vi "BasicExampleWithIFw.vi"() -> ()   [LabVIEW 2015]
uses:
  QuadEnc/Output.ctl
  <vilib>/Platform/TimedLoop/XDataNode/timing_clust.ctl
  <vilib>/Platform/TimedLoop/XDataNode/nitl_modes.ctl
  <vilib>/Platform/TimedLoop/XDataNode/wakeup.ctl
  <vilib>/rvi/Emulation/niFpgaSctlEmulationGetInTimedLoop.vi
  <vilib>/rvi/Emulation/niFpgaEmulationReportErrorSimple.vi
  <vilib>/rvi/Emulation/niFpgaGetClockAttributes.vi
  <vilib>/rvi/Emulation/niFpgaCriticalErrorInLSC.vi
  <vilib>/rvi/eio/common/nirviEmuTemplateMethod_errors.vi
  <vilib>/Platform/TimedLoop/XDataNode/XDataNode.xnode
  <vilib>/eio/EIONode/EIONode.xnode
  <instrlib>/_niInstr/Instruction Framework/v1/FPGA/Top Level Bus/Register Configuration/Register Configuration.lvclass
  <vilib>/Platform/TimedLoop/XDataNode/XDNodeRunTimeDep.lvlib
  QuadEnc/AddressSpace.lvclass
  QuadEnc/QuadEnc.lvlib
  <instrlib>/_niInstr/FIFO Register Bus/v1/FPGA/niInstr FIFO Register Bus v1 FPGA.lvclass
panel:
  in  "fifo reg bus ctrl 0":u32
  out "fifo reg bus status 0":u32
  out "fifo reg bus data 0":u64
  in  "reset":bool
  out "AbsPosition":i32
  out "RevPosition":i32
  out "CW_direction":bool
  out "Output":T1
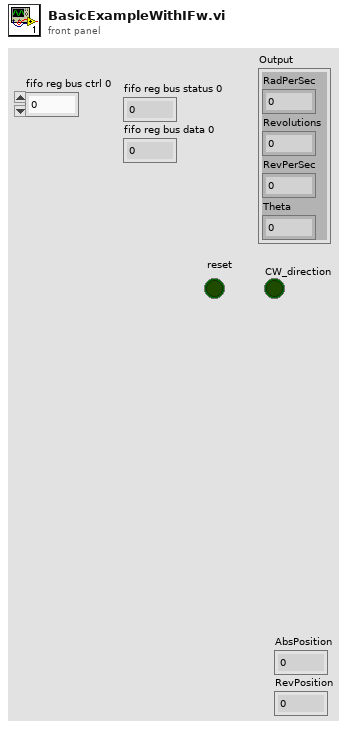
[diagram p1: front panel]
types:
  T1 = typedef "QuadEnc.lvlib/Output.ctl" = cluster{"RadPerSec":sgl, "Revolutions":sgl, "RevPerSec":sgl, "Theta":sgl}
  T2 = typedef "XDNodeRunTimeDep.lvlib/timing_clust.ctl" = cluster{"Expected End [f-1]":u64, "Actual End [f-1]":u64, "Finished Late? [f-1]":bool, "Expected End [i-1]":u64, "Actual End [i-1]":u64, "Finished Late? [i-1]":bool, "Expected Start [i]":u64, "Actual Start [i]":u64, "Expected Start [f]":u64, "Actual Start [f]":u64, "Source Name":string, "Structure Name":string, "Period":i64, "Deadline":i64, "Offset":i64, "Start":i64, "Priority":i32, "Timeout":i32, "Mode":T3, "Wakeup Reason":T4, "Error":errorcluster, "Source Type":string, "Secondary Source Type":string, "Global End Time":u64, "Global Start Time":u64, "Frame Duration":u64, "Iteration Duration":u64, "Assigned CPU":i32, "I/O Scan Engine Mode":u32}
  T3 = typedef "XDNodeRunTimeDep.lvlib/nitl_modes.ctl" = enum32{"No Change", "Process missed periods, maintain original phase", "Discard missed periods, maintain original phase", "Process missed periods, ignore original phase", "Discard missed periods, ignore original phase"}
  T4 = typedef "XDNodeRunTimeDep.lvlib/wakeup.ctl" = enum32{"Normal", "Aborted", "Asynchronous wakeup", "Timing source error", "Timed loop error", "Timeout"}
  T5 = typedef "QuadEnc.lvlib/Parameters.ctl" = cluster{"ReversePolarity":refnum<k21>, "dTPerSec":refnum<k21>, "RevPerPulse":refnum<k21>, "dT":refnum<k21>}
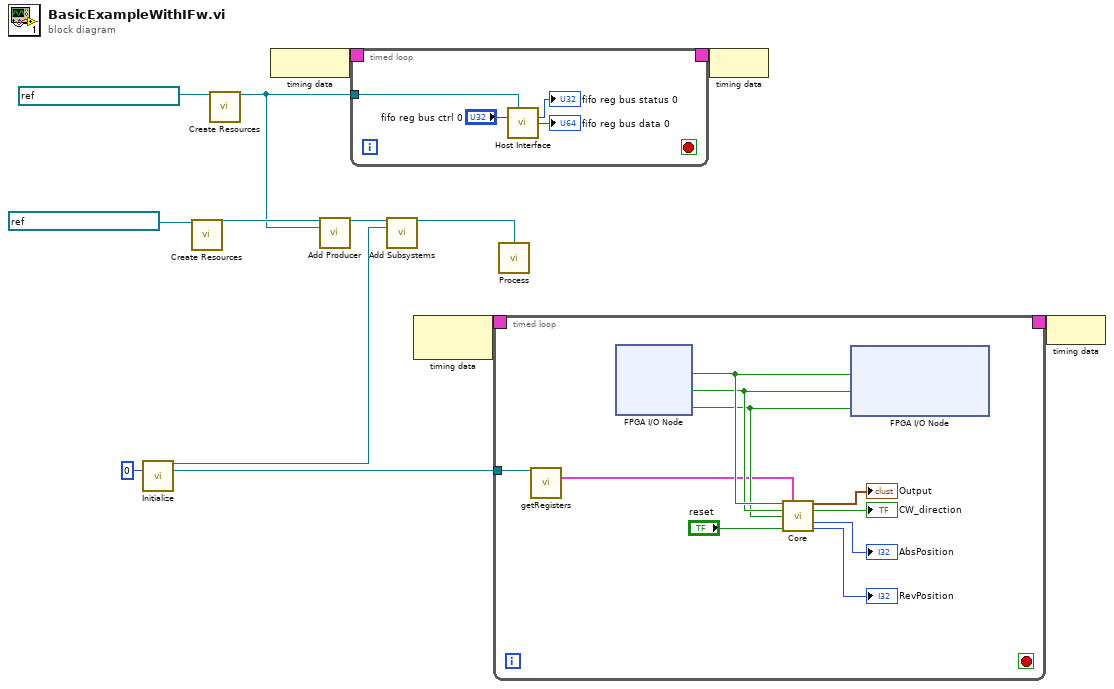
[diagram p0: block diagram]
diagram:
  n1 = call "Initialize.vi"("instance"=u8 0) -> ("subsystem"=w6:refnum<class "Single Address Space Collection.lvclass">, "AddressSpace"=w5:refnum<class "AddressSpace.lvclass">)  [unwired: 13 in]
  n2 = call <instrlib>:"Create Resources.vi"("register clock"=refnum<k21> "40 MHz Onboard Clock") -> ("register configuration"=w13:refnum<class "Register Configuration.lvclass">)  [unwired: 14 in]
  n3 = call <instrlib>:"Create Resources.vi"("instruction fifo"=refnum<k21> "reg.host instruction fifo 0") -> ("fifo register bus"=w1:refnum<class "niInstr FIFO Register Bus v1 FPGA.lvclass">)  [unwired: 14 in]
  n4 = node-c288() -> (w4:T2)
  n5 = call <instrlib>:"Add Producer.vi"("register configuration in"=w13, "instruction producer"=w1) -> ("register configuration out"=w11:refnum<class "Register Configuration.lvclass">)  [unwired: 13 in]
  n6 = timed-loop {
    timing: w4 -> [_]
    timing-out: [_] -> w3
    tunnel: w1 -> [w17]
    stop <- _ stop-if-true
    n7 = call <instrlib>:"Host Interface.vi"("fifo register bus"=w17, "fifo reg bus ctrl 0"="fifo reg bus ctrl 0") -> ("fifo reg bus status 0"=→"fifo reg bus status 0":u32, "fifo reg bus data 0"=→"fifo reg bus data 0":u64)  [unwired: 12 in]
  }
  n8 = call <instrlib>:"Add Subsystems.vi"("register configuration in"=w11, "subsystems"=w6) -> ("register configuration out"=w10:refnum<class "Register Configuration.lvclass">)  [unwired: 13 in]
  n9 = node-c288() -> (w8:T2)  [unwired: 1 in]
  n10 = timed-loop {
    timing: w8 -> [_]
    timing-out: [_] -> w7
    tunnel: w5 -> [w21]
    stop <- _ stop-if-true
    n11 = call "getRegisters.vi"("AddressSpace in"=w21) -> ("Parameters"=w20:T5)  [unwired: 13 in, 1 out]
    n12 = xnode "FPGA I/O Node"() -> ("Enc_A"=w29:bool, "Enc_B"=w28:bool, "Enc_Z"=w27:bool)  [unwired: 3 in, 3 out]
    n13 = call "Core.vi"("A"=w29, "Parameters"=w20, "B"=w28, "Z"=w27, "reset"="reset") -> ("Output"=→"Output":T1, "CW_direction"=→"CW_direction":bool, "AbsPosition"=→"AbsPosition":i32, "RevPosition"=→"RevPosition":i32)  [unwired: 7 in]
    n14 = xnode "FPGA I/O Node"("GPIC/LVTTL/DIO3"=w29, "GPIC/LVTTL/DIO4"=w28, "GPIC/LVTTL/DIO5"=w27) -> ()  [unwired: 3 in, 3 out]
  }
  n15 = call <instrlib>:"Process.vi"("register configuration"=w10) -> ()  [unwired: 15 in]
  n16 = node-c288(w3) -> ()
  n17 = node-c288(w7) -> ()
